vi "Apply cRIO voltage and hold.vi"() -> ()   [LabVIEW 2020]
panel:
  in  "stop":bool
  out "error out":errorcluster
  in  "Voltage":dbl
  in  "AO Channel":string(combo)="AO0"
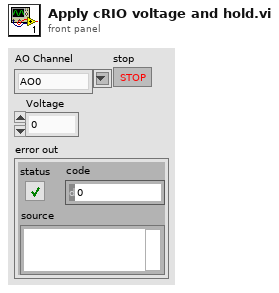
[diagram p1: front panel]
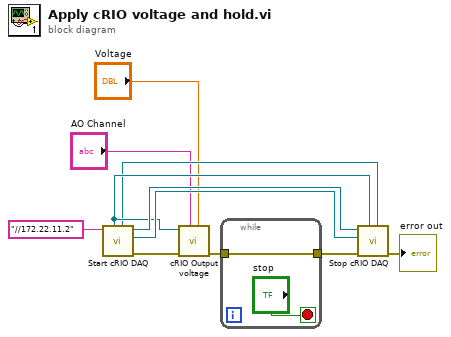
[diagram p0: block diagram]
diagram:
  n1 = call "Start cRIO DAQ.vi"("cRIO IP"="//172.22.11.2") -> ("error out"=w6:errorcluster, "vi reference"=w9:refnum<vi>, "application reference"=w10:refnum<vi>, "DAQ_AI_Reader endpoint"=w7:refnum<k21>, "DAQ_CMD_Writer endpoint"=w8:refnum<k21>)  [unwired: 6 in]
  n2 = call "cRIO Output voltage.vi"("Voltage"="Voltage", "AO Channel"="AO Channel", "error in (no error)"=w6, "DAQ_CMD_Writer endpoint"=w8) -> ("error out"=w3:errorcluster)  [unwired: 6 in, 1 out]
  n3 = while {
    tunnel: w3 -> [w13]
    tunnel: [w13] -> w2
    stop <- "stop" stop-if-true
  }
  n4 = call "Stop cRIO DAQ.vi"("DAQ_AI_Reader endpoint"=w7, "DAQ_CMD_Writer endpoint"=w8, "error in (no error)"=w2, "VI reference"=w9, "application reference"=w10) -> ("error out"=→"error out":errorcluster)  [unwired: 6 in]
